vi "Init.vi"(8 "error in (no error)":errorcluster, 11 "SOL Server":refnum<class "SOL-Server.lvclass">) -> (0 "error out":errorcluster, 3 "Error Logger out":refnum<class "Error Logger.lvclass">)   [LabVIEW 2020, in "Summer of LabVIEW.lvlib" / "Error Logger.lvclass"]
uses:
  Error Logger.lvclass
  Error Logger.lvclass/Error Logger.ctl
  SOL-Server/SOL-Server.lvclass
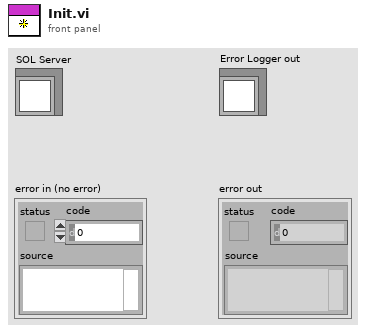
[diagram p1: front panel]
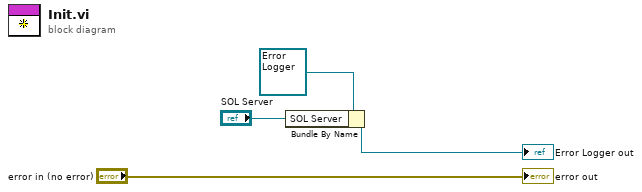
[diagram p0: block diagram]
diagram:
  n1 = Bundle By Name(cluster=refnum<class "Error Logger.lvclass"> refnum ("Error Logger in"), "SOL Server"="SOL Server") -> (→"Error Logger out":refnum<class "Error Logger.lvclass">)
  "error out" <- "error in (no error)"
